vi "Populate Event Register.vi"(8 "error in (no error)":errorcluster, 10 "User Events":refnum<user-event>, 11 "Event Registration Refnum":refnum<event-registration>) -> (0 "error out":errorcluster)   [LabVIEW 2013, in "main.lvlib"]
uses:
  main.lvlib
  Components/Dependencies.llb/Exit Event Ref.ctl
  Controls/Reference AE Control.ctl
  Components/Dependencies.llb/TLB_Dependencies.lvlib
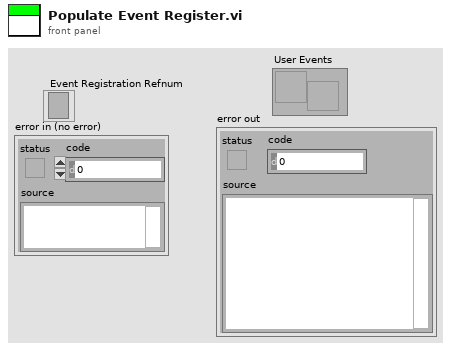
[diagram p1: front panel]
types:
  T1 = typedef "main.lvlib/Reference AE Control.ctl" = enum16{"Initialize", "Set Menu", "Set Profile", "Set Configuration", "Set Configuration_old", "Set Configuration_new", "Set Configuration Method", "Set Acquisition", "Set Data", "Set Journal", "Get"}
  T2 = typedef "main.lvlib/Reference Cluster.ctl" = cluster{"Menu":cluster{"References":cluster{"Stop Acq":refnum<vi>, "MenuExit":refnum<vi>, "MenuStartADC":refnum<vi>, "PersonalInfoString":refnum<vi>, "Profile":refnum<vi>, "Configuration":refnum<vi>, "Acquisition":refnum<vi>, "Data":refnum<vi>, "Journal":refnum<vi>}}, "Profile":cluster{"References":cluster{"Search Patient ID":refnum<vi>, "Name":refnum<vi>, "CommentStr":refnum<vi>, "Listbox Patient ID":refnum<vi>, "ListboxDoctor":refnum<vi>, "ListboxOperator":refnum<vi>, "HospitalName":refnum<vi>, "HospitalDepartment":refnum<vi>, "HospitalAddress":refnum<vi>, "EditHospInfo":refnum<vi>, "Add Patient ID Btn":refnum<vi>, "Query Worklist":refnum<vi>}}, "Configuration":cluster{"References":cluster{"ListboxMeasurementArea":refnum<vi>, "ListboxMeasurementTechnique":refnum<vi>, "ListboxMeasurementMeth":refnum<vi>, "ListboxRightSegmentNr":refnum<vi>, "ListboxLeftSegmentNr":refnum<vi>, "HeightAdjustmentInt":refnum<vi>, "PalpationRight":refnum<vi>, "PalpationLeft":refnum<vi>, "ActivityBox":refnum<vi>}, "New method":cluster{"AddNewMeasurementBtn":refnum<vi>, "Left Time Table":refnum<vi>, "Right Time Table":refnum<vi>}, "Old method":cluster{"LeftArmPressureTable":refnum<vi>, "RightArmPressureTable":refnum<vi>, "SaveArmPressureBtn":refnum<vi>, "Puls":refnum<vi>, "TempTwo":refnum<vi>, "TempOne":refnum<vi>}, "Method":string}, "Acquisition":cluster{"References":cluster{"SegmentAcqString":refnum<vi>, "RingActGraph":refnum<vi>}}, "Data":cluster{"References":cluster{"cmString":refnum<vi>, "AdjustedHeight":refnum<vi>, "Menu":refnum<vi>, "Tangent On/Off":refnum<vi>, "FilterControl":refnum<vi>}}, "Journal":cluster{"References":cluster{"ReportSelection":refnum<vi>, "Data":refnum<vi>, "GenerateReport":refnum<vi>, "Menu":refnum<vi>, "Send To PACS":refnum<vi>}}}
  T3 = cluster{"Stop Acq":refnum<vi>, "MenuExit":refnum<vi>, "MenuStartADC":refnum<vi>, "PersonalInfoString":refnum<vi>, "Profile":refnum<vi>, "Configuration":refnum<vi>, "Acquisition":refnum<vi>, "Data":refnum<vi>, "Journal":refnum<vi>}
  T4 = cluster{"Search Patient ID":refnum<vi>, "Name":refnum<vi>, "CommentStr":refnum<vi>, "Listbox Patient ID":refnum<vi>, "ListboxDoctor":refnum<vi>, "ListboxOperator":refnum<vi>, "HospitalName":refnum<vi>, "HospitalDepartment":refnum<vi>, "HospitalAddress":refnum<vi>, "EditHospInfo":refnum<vi>, "Add Patient ID Btn":refnum<vi>, "Query Worklist":refnum<vi>}
  T5 = cluster{"ListboxMeasurementArea":refnum<vi>, "ListboxMeasurementTechnique":refnum<vi>, "ListboxMeasurementMeth":refnum<vi>, "ListboxRightSegmentNr":refnum<vi>, "ListboxLeftSegmentNr":refnum<vi>, "HeightAdjustmentInt":refnum<vi>, "PalpationRight":refnum<vi>, "PalpationLeft":refnum<vi>, "ActivityBox":refnum<vi>}
  T6 = cluster{"SegmentAcqString":refnum<vi>, "RingActGraph":refnum<vi>}
  T7 = cluster{"cmString":refnum<vi>, "AdjustedHeight":refnum<vi>, "Menu":refnum<vi>, "Tangent On/Off":refnum<vi>, "FilterControl":refnum<vi>}
  T8 = cluster{"ReportSelection":refnum<vi>, "Data":refnum<vi>, "GenerateReport":refnum<vi>, "Menu":refnum<vi>, "Send To PACS":refnum<vi>}
  T9 = cluster{"LeftArmPressureTable":refnum<vi>, "RightArmPressureTable":refnum<vi>, "SaveArmPressureBtn":refnum<vi>, "Puls":refnum<vi>, "TempTwo":refnum<vi>, "TempOne":refnum<vi>}
  T10 = cluster{"AddNewMeasurementBtn":refnum<vi>, "Left Time Table":refnum<vi>, "Right Time Table":refnum<vi>}
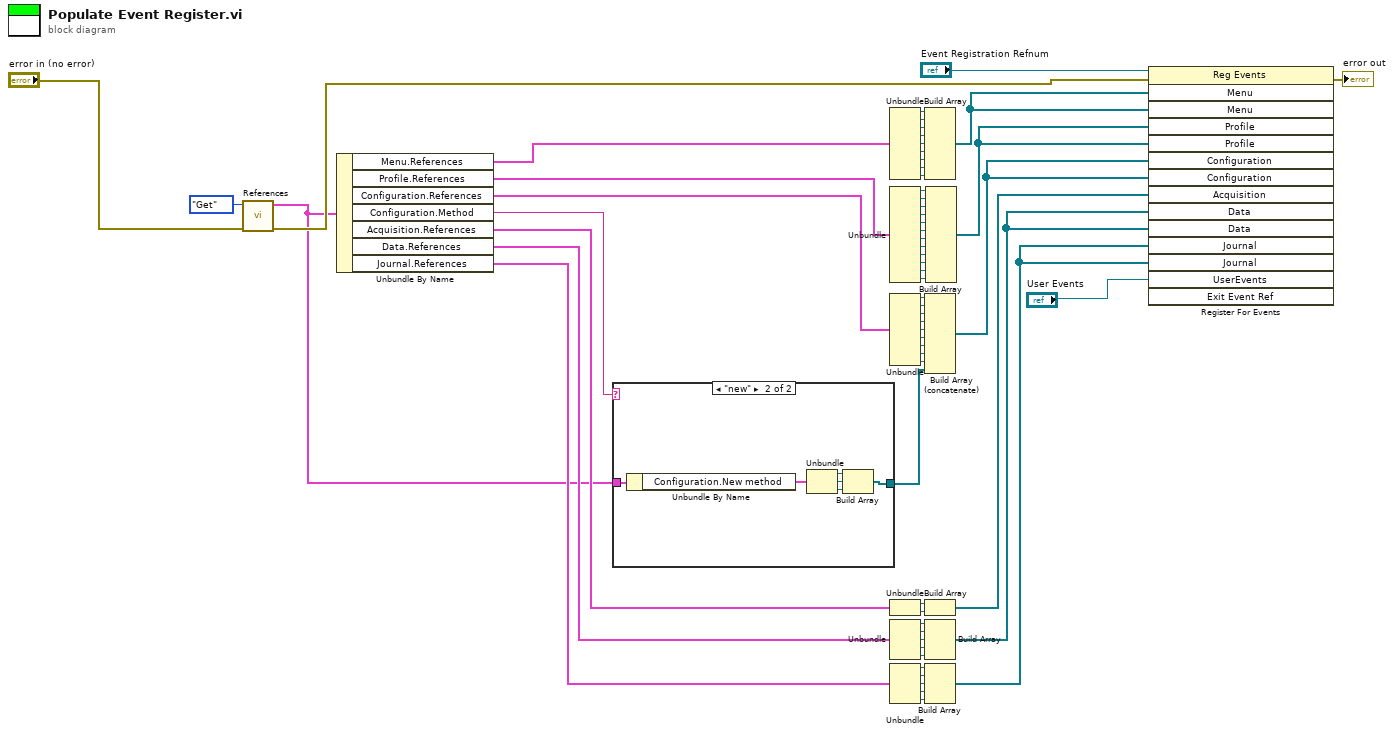
[diagram p0: block diagram]
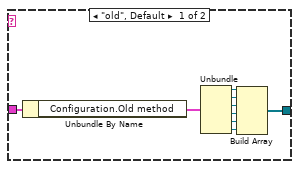
[diagram p2: hidden frame]
diagram:
  n1 = call "References.vi"("error in"="error in (no error)", "Reference AE Control"=Reference_AE_Control."Get") -> ("error out"=w6:errorcluster, "Cluster out"=w2:T2)  [unwired: 8 in]
  n2 = Unbundle By Name(w2) -> ("Menu.References"=w61:T3, "Profile.References"=w54:T4, "Configuration.References"=w41:T5, "Configuration.Method"=w3:string, "Acquisition.References"=w30:T6, "Data.References"=w26:T7, "Journal.References"=w19:T8)
  n3 = case shown="\"new\"" w3 {
    tunnel: w2 -> [w72 w74]
    tunnel: [w64 w73] -> w1
    frame "old", Default {
      n4 = Unbundle By Name(w72) -> ("Configuration.Old method"=w71:T9)
      n5 = Unbundle(w71) -> ("LeftArmPressureTable"=w70:refnum<vi>, "RightArmPressureTable"=w69:refnum<vi>, "SaveArmPressureBtn"=w68:refnum<vi>, "Puls"=w67:refnum<vi>, "TempTwo"=w66:refnum<vi>, "TempOne"=w65:refnum<vi>)
      n6 = Build Array(w70, w69, w68, w67, w66, w65) -> (w64:refnum<vi>[])
    }
    frame "new" {
      n7 = Unbundle By Name(w74) -> ("Configuration.New method"=w78:T10)
      n8 = Unbundle(w78) -> ("AddNewMeasurementBtn"=w77:refnum<vi>, "Left Time Table"=w76:refnum<vi>, "Right Time Table"=w75:refnum<vi>)
      n9 = Build Array(w77, w76, w75) -> (w73:refnum<vi>[])
    }
  }
  n10 = Unbundle(w61) -> ("Stop Acq"=w60:refnum<vi>, "MenuExit"=w59:refnum<vi>, "MenuStartADC"=w58:refnum<vi>, "PersonalInfoString"=w57:refnum<vi>, "Profile"=w56:refnum<vi>, "Configuration"=w12:refnum<vi>, "Acquisition"=w11:refnum<vi>, "Data"=w10:refnum<vi>, "Journal"=w9:refnum<vi>)
  n11 = Unbundle(w54) -> ("Search Patient ID"=w53:refnum<vi>, "Name"=w52:refnum<vi>, "CommentStr"=w51:refnum<vi>, "Listbox Patient ID"=w50:refnum<vi>, "ListboxDoctor"=w49:refnum<vi>, "ListboxOperator"=w48:refnum<vi>, "HospitalName"=w47:refnum<vi>, "HospitalDepartment"=w46:refnum<vi>, "HospitalAddress"=w45:refnum<vi>, "EditHospInfo"=w44:refnum<vi>, "Add Patient ID Btn"=w43:refnum<vi>, "Query Worklist"=w4:refnum<vi>)
  n12 = Unbundle(w41) -> ("ListboxMeasurementArea"=w40:refnum<vi>, "ListboxMeasurementTechnique"=w39:refnum<vi>, "ListboxMeasurementMeth"=w38:refnum<vi>, "ListboxRightSegmentNr"=w37:refnum<vi>, "ListboxLeftSegmentNr"=w36:refnum<vi>, "HeightAdjustmentInt"=w35:refnum<vi>, "PalpationRight"=w34:refnum<vi>, "PalpationLeft"=w33:refnum<vi>, "ActivityBox"=w32:refnum<vi>)
  n13 = Unbundle(w30) -> ("SegmentAcqString"=w29:refnum<vi>, "RingActGraph"=w28:refnum<vi>)
  n14 = Unbundle(w26) -> ("cmString"=w25:refnum<vi>, "AdjustedHeight"=w24:refnum<vi>, "Menu"=w23:refnum<vi>, "Tangent On/Off"=w22:refnum<vi>, "FilterControl"=w21:refnum<vi>)
  n15 = Unbundle(w19) -> ("ReportSelection"=w18:refnum<vi>, "Data"=w17:refnum<vi>, "GenerateReport"=w16:refnum<vi>, "Menu"=w15:refnum<vi>, "Send To PACS"=w5:refnum<vi>)
  n16 = Build Array(w60, w59, w58, w57, w56, w12, w11, w10, w9) -> (w55:refnum<vi>[])
  n17 = Build Array (concatenate)(w40, w39, w38, w37, w36, w35, w34, w33, w32, w1) -> (w31:refnum<vi>[])
  n18 = Build Array(w29, w28) -> (w27:refnum<vi>[])
  n19 = Build Array(w25, w24, w23, w22, w21) -> (w20:refnum<vi>[])
  n20 = Build Array(w18, w17, w16, w15, w5) -> (w14:refnum<vi>[])
  n21 = Build Array(w53, w52, w51, w50, w49, w48, w47, w46, w45, w44, w43, w4) -> (w42:refnum<vi>[])
  n22 = register-events(reference="Event Registration Refnum", error in=w6, w55, w55, w42, w42, w31, w31, w27, w20, w20, w14, w14, "User Events") -> (error out=→"error out":errorcluster)  [unwired: 1 in, 1 out]
